vi "DEMO AC and PNA.vi"() -> ()   [LabVIEW 2017]
uses:
  Classes/N5222A PNA/N5222A PNA.lvclass
  Classes/ArrayController/ArrayController.lvclass
  Classes/ArrayController/ACConfig.ctl
  Classes/Sequence/SequenceSubvis/PolarizationSelect.ctl
  Classes/Sequence/SequenceSubvis/RF Direction.ctl
  Classes/Datalog/DatalogSubvis/SearchableTag.ctl
  Classes/Datalog/DataLog.lvclass
panel:
  out "error out":errorcluster
  out "AC Temp, deg C":dbl
  in  "AC Reset (True)":bool
  in  "AC d Command":T1
  in  "AC Config":T4={"ACIPAddress"="192.168.1.110", "timeout ms"=1000, "AC (Dest.) port"=0, "Enable"=FALSE}
  out ".csv file":string
  out "Cal Files by name":string[](array[string])
  in  "N5222A Cfg":T5={"ResourceName"="PNA", "Enable"=TRUE, "Channel"=1, "CalFileName"="CalSet_Peisangtsai_040315_apar_-10dBm", "MeasName"="SxxMeas%d", "TempDatFile"="APARscratch.csv", "Power, dBm"=-30.0, "NumPoints"=201, "Start Freq, Hz"=5000000000.0, "Stop Freq, Hz"=6000000000.0} {"Stop Freq, Hz" format="%_3p"; "Start Freq, Hz" format="%_3p"}
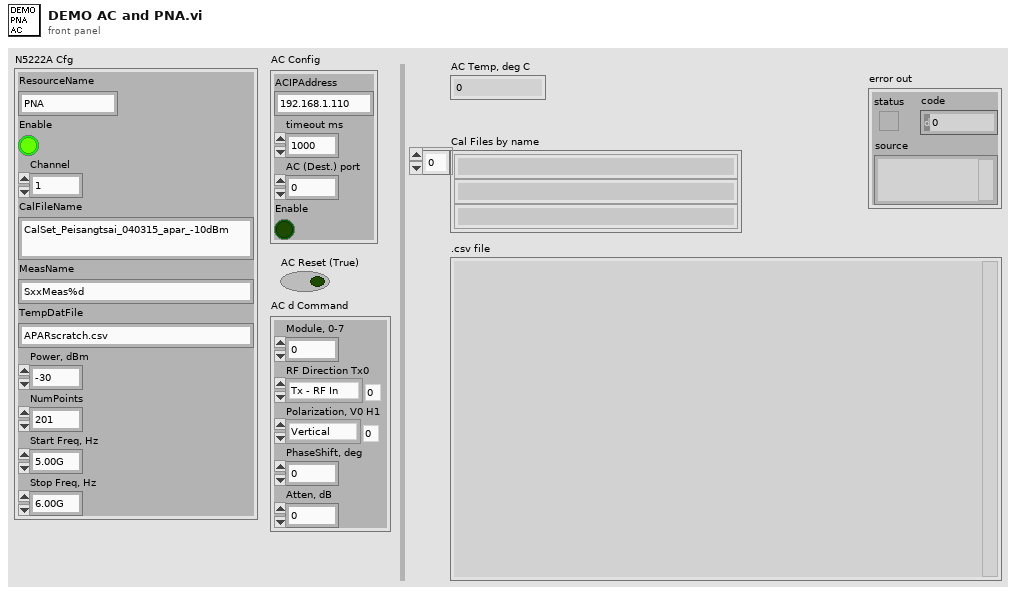
[diagram p1: front panel]
types:
  T1 = typedef "DataLog.lvclass/SearchableTag.ctl" = cluster{"Module, 0-7":i32, "RF Direction Tx0":T2, "Polarization, V0 H1":T3, "PhaseShift, deg":dbl, "Atten, dB":dbl}
  T2 = typedef "RF Direction.ctl" = enum16{"Tx - RF In", "Rx - RF Out"}
  T3 = typedef "PolarizationSelect.ctl" = enum16{"Vertical", "Horizontal"}
  T4 = typedef "ACConfig.ctl" = cluster{"ACIPAddress":string, "timeout ms":i32, "AC (Dest.) port":u16, "Enable":bool}
  T5 = cluster{"ResourceName":string, "Enable":bool, "Channel":i32, "CalFileName":string, "MeasName":string, "TempDatFile":string, "Power, dBm":dbl, "NumPoints":i32, "Start Freq, Hz":dbl, "Stop Freq, Hz":dbl}
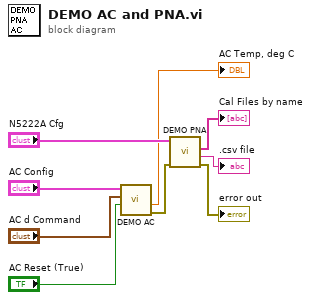
[diagram p0: block diagram]
diagram:
  n1 = call "DEMO AC.vi"("Reset (True)"="AC Reset (True)", "SectionProperties"="AC d Command", "AC Config"="AC Config") -> ("error out"=w2:errorcluster, "Temp, deg C"=→"AC Temp, deg C":dbl)  [unwired: 7 in]
  n2 = call "DEMO PNA.vi"("error in (no error)"=w2, "N5222A Cfg"="N5222A Cfg") -> ("error out"=→"error out":errorcluster, ".csv file"=→".csv file":string, "Cal Files by name"=→"Cal Files by name":string[])  [unwired: 7 in]
